vi "Inc_Switch.vi"(10 "Numeric in":i32, 11 "Ele_At_Pos":bool) -> (3 "Numeric out":i32)   [LabVIEW 2014]
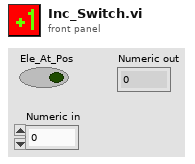
[diagram p1: front panel]
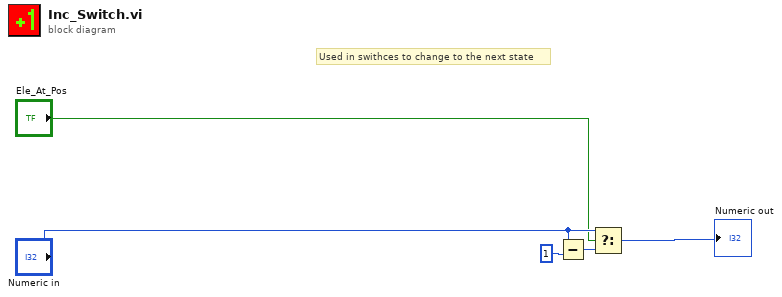
[diagram p0: block diagram]
diagram:
  # "Used in swithces to change to the next state"
  n1 = Subtract(x="Numeric in", y=1) -> (x-y=w3:i32)
  n2 = Select(t="Numeric in", s="Ele_At_Pos", f=w3) -> (s? t:f=→"Numeric out":i32)
